vi "__deleteItemFromRoom.vi"(8 "room_device_type":T1, 9 "devicesToRemove":string[](array[string]), 10 "roomGUID":string, 11 "Room-API In":refnum<class "Room-API.lvclass">) -> (0 "error out":errorcluster, 3 "Room-API out":refnum<class "Room-API.lvclass">)   [LabVIEW 2020, in "Room-API.lvclass"]
uses:
  Room-API.lvclass
  __room_device_type.ctl
  Room-API.lvclass/Room-API.ctl
  <userlib>/_OpenG.lib/array/array.llb/Filter 1D Array (String)__ogtk.vi
  <vilib>/ErrorRing/Error Ring.xnode
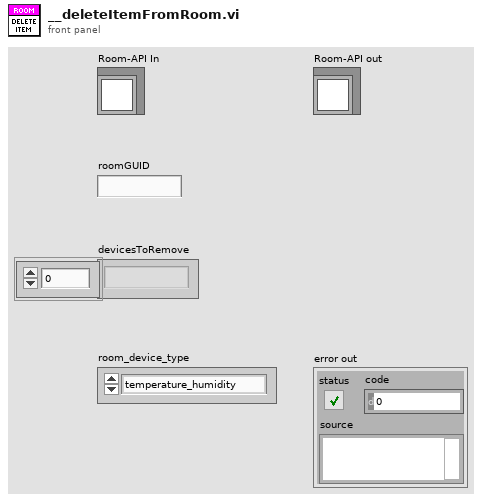
[diagram p1: front panel]
types:
  T1 = typedef "Room-API.lvclass/__room_device_type.ctl" = enum16{"temperature_humidity", "bond", "hue"}
  T2 = typedef "Room-API.lvclass/Single Room.ctl" = cluster{"name":string, "temperature_humidity":string[], "bond":string[], "hue":string[]}
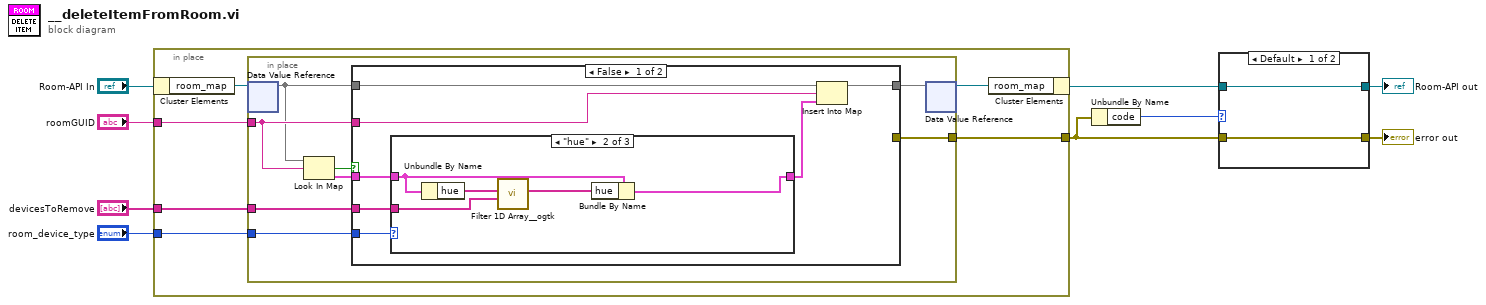
[diagram p0: block diagram]
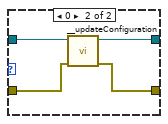
[diagram p2: hidden frame]
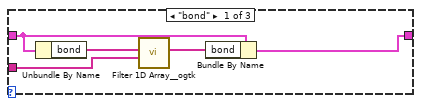
[diagram p3: hidden frame]
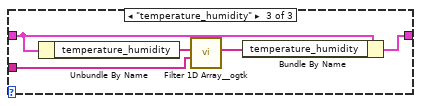
[diagram p4: hidden frame]
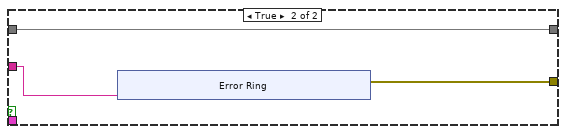
[diagram p5: hidden frame]
diagram:
  n1 = in-place {
    in-place-border: "devicesToRemove" -> [w15]
    in-place-border: "roomGUID" -> [w14]
    in-place-border: "room_device_type" -> [w13]
    in-place-border: [w12] -> w2
    n2 = in-place-cluster #1("Room-API In") -> ("room_map"=w11:refnum<data-value>)
    n3 = in-place {
      in-place-border: w15 -> [w21]
      in-place-border: w14 -> [w20]
      in-place-border: w13 -> [w19]
      in-place-border: [w18] -> w12
      n4 = in-place-dvr #2(w11) -> (w17:map{string, T2})  [unwired: 1 out]
      n5 = Look In Map(map=w17, key=w20) -> (key not found?=w23:bool, value=w22:T2)  [unwired: 1 in]
      n6 = case shown="False" w23 {
        tunnel: w22 -> [w25 _]
        tunnel: w17 -> [w30 w48]
        tunnel: [w29 w48] -> w16
        tunnel: w21 -> [w26 _]
        tunnel: w20 -> [w28 w47]
        tunnel: w19 -> [w27 _]
        tunnel: [_ w46] -> w18
        frame False {
          n7 = case shown="\"hue\"" w27 {
            tunnel: w26 -> [w31 w37 w42]
            tunnel: w25 -> [w35 w40 w45]
            tunnel: [w34 w39 w44] -> w24
            frame "bond" {
              n8 = Unbundle By Name(w35) -> ("bond"=w33:string[])
              n9 = call-poly <userlib>:"Filter 1D Array__ogtk.vi"("items to filter"=w31, "array"=w33) -> ("filtered array"=w32:string[])  [unwired: 4 in, 1 out]
              n10 = Bundle By Name(cluster=w35, "bond"=w32) -> (w34:T2)
            }
            frame "hue" {
              n11 = Unbundle By Name(w40) -> ("hue"=w38:string[])
              n12 = call-poly <userlib>:"Filter 1D Array__ogtk.vi"("items to filter"=w37, "array"=w38) -> ("filtered array"=w36:string[])  [unwired: 4 in, 1 out]
              n13 = Bundle By Name(cluster=w40, "hue"=w36) -> (w39:T2)
            }
            frame "temperature_humidity" {
              n14 = Unbundle By Name(w45) -> ("temperature_humidity"=w43:string[])
              n15 = call-poly <userlib>:"Filter 1D Array__ogtk.vi"("items to filter"=w42, "array"=w43) -> ("filtered array"=w41:string[])  [unwired: 4 in, 1 out]
              n16 = Bundle By Name(cluster=w45, "temperature_humidity"=w41) -> (w44:T2)
            }
          }
          n17 = Insert Into Map(map in=w30, key=w28, value=w24) -> (map out=w29:map{string, T2})  [unwired: 2 out]
        }
        frame True {
          n18 = xnode "Error Ring"("parameter 0"=w47) -> ("error out"=w46:errorcluster)
        }
      }
      n19 = in-place-dvr #2(w16) -> (w10:refnum<data-value>)  [unwired: 1 out]
    }
    n20 = in-place-cluster #1("room_map"=w10) -> (w5:refnum<class "Room-API.lvclass">)
  }
  n21 = Unbundle By Name(w2) -> ("code"=w1:i32)
  n22 = case shown="Default" w1 {
    tunnel: w5 -> [w55 w59]
    tunnel: [w55 w58] -> w4
    tunnel: w2 -> [w54 w57]
    tunnel: [w54 w56] -> w3
    frame Default {
    }
    frame 0 {
      n23 = call "__updateConfiguration.vi"("error in (no error)"=w57, "Room-API in"=w59) -> ("error out"=w56:errorcluster, "Room-API out"=w58:refnum<class "Room-API.lvclass">)  [unwired: 8 in]
    }
  }
  "error out" <- w3
  "Room-API out" <- w4
